vi "CTI passwords custom error codes.vi"(4 "Add source? (T)":bool=TRUE, 5 "error index":i32) -> (0 "error out":errorcluster={"status"=FALSE, "code"=8000, "source"=""})   [LabVIEW 2013]
doc: "Use this vi for defining all custom error codes and strings for CTI standard password VIs.\n\nKeep all custom error codes and strings in this vi's front panel array and save as default. Never delete items in array (just don't use if obsolete).\n\nError index input is required."
panel:
  in  "Custom errors":cluster{"code":i32, "string":string}[](array[cluster])=[{"code"=8000, "string"="Error reading password file or no users in list."}]
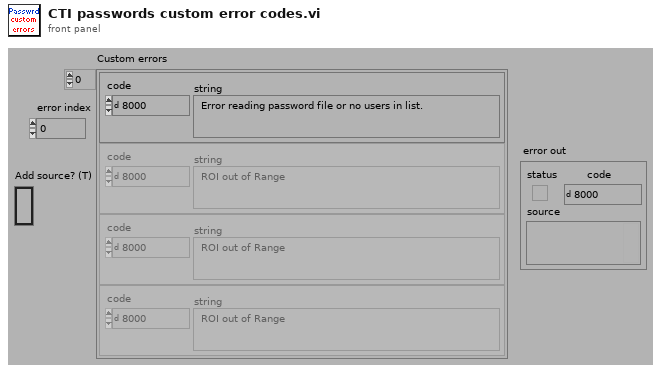
[diagram p1: front panel]
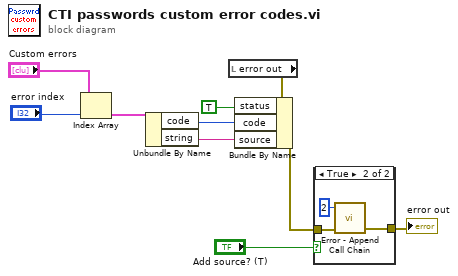
[diagram p0: block diagram]
diagram:
  n1 = Index Array(array="Custom errors", index="error index") -> (element=w7:cluster{"code":i32, "string":string})
  n2 = Unbundle By Name(w7) -> ("code"=w6:i32, "string"=w5:string)
  n3 = local read "error out"() -> (w8:errorcluster)
  n4 = Bundle By Name(cluster=w8, "status"=TRUE ("Bundle Element"), "code"=w6, "source"=w5) -> (w2:errorcluster)
  n5 = case shown="True" "Add source? (T)" {
    tunnel: w2 -> [w11 w14]
    tunnel: [w11 w13] -> w1
    frame False {
    }
    frame True {
      n6 = call "Error - Append Call Chain.vi"("error in (no error)"=w14, "Layers Up (1)"=2) -> ("error out"=w13:errorcluster)  [unwired: 3 out]
    }
  }
  "error out" <- w1
